vi "SetGetModuleList.vi"(7 "Set? (f)":bool, 11 "ModuleList":string[](array[string])) -> (3 "ModuleList":string[](array[string]))   [LabVIEW 2014, in "Test.lvclass"]
uses:
  Test.lvclass
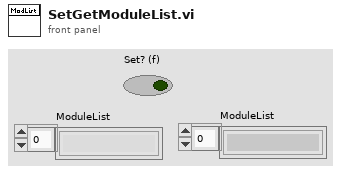
[diagram p1: front panel]
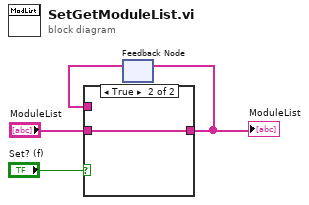
[diagram p0: block diagram]
diagram:
  n1 = feedback #1() -> (w1:string[])  [unwired: 1 in]
  n2 = case shown="True" "Set? (f)" {
    tunnel: [w5 w6] -> w3
    tunnel: "ModuleList" -> [_ w6]
    tunnel: w1 -> [w5 _]
    frame False {
    }
    frame True {
    }
  }
  "ModuleList" <- w3
  n3 = feedback-in #1(w3) -> ()
